vi "2.Réservoir_GJE.vi"() -> ()   [LabVIEW 2018]
panel:
  in  "Consigne":i16(slide) min=0 max=1000 scale=0.0..1000.0
  in  "Débit":i8(slide)=1 min=1 max=10 scale=1.0..10.0
  in  "stop":bool
  out "Tank":i16(slide) scale=0.0..1000.0
  # "1/s"
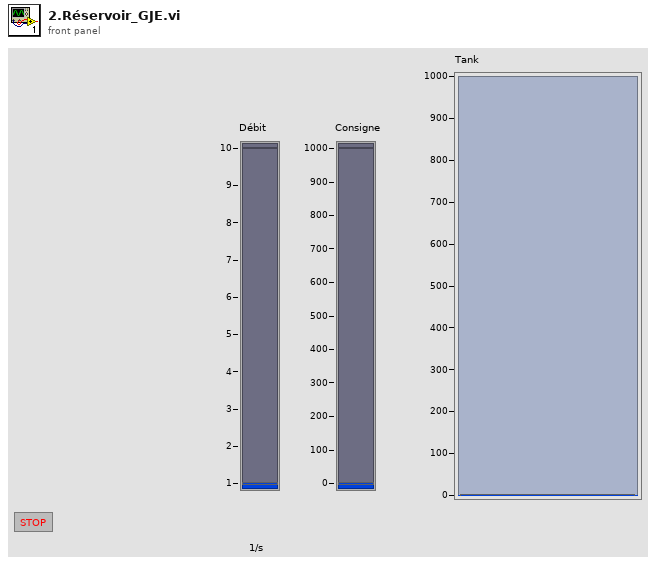
[diagram p1: front panel]
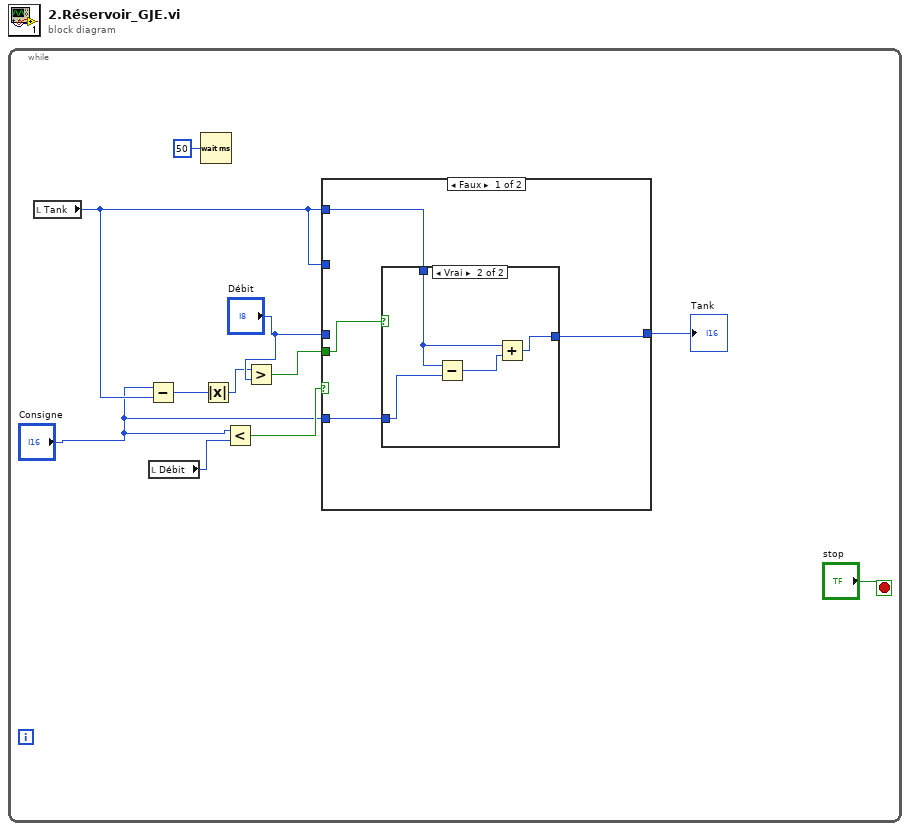
[diagram p0: block diagram]
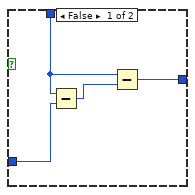
[diagram p2: hidden frame]
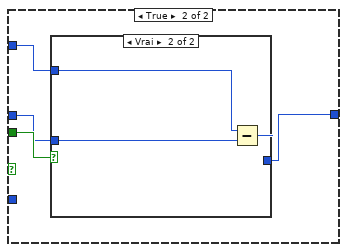
[diagram p3: hidden frame]
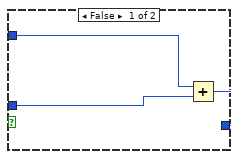
[diagram p4: hidden frame]
diagram:
  n1 = while {
    stop <- "stop" stop-if-true
    n2 = local read "Tank"() -> (w4:i16)
    n3 = Subtract(x="Consigne", y=w4) -> (x-y=w8:i16)
    n4 = local read "Débit"() -> (w1:i8)
    n5 = Wait (ms)(milliseconds to wait=u32 50) -> ()  [unwired: 1 out]
    n6 = Absolute Value(x=w8) -> (abs(x)=w6:i16)
    n7 = Less?(x="Consigne", y=w1) -> (x < y?=w3:bool)
    n8 = Greater?(x=w6, y="Débit") -> (0:w9:bool)
    n9 = case shown="Faux" w3 {
      tunnel: w9 -> [w13 w27]
      tunnel: w4 -> [_ w26]
      tunnel: "Débit" -> [_ w25]
      tunnel: [w12 w24] -> w5
      tunnel: w4 -> [w15 _]
      tunnel: "Consigne" -> [w14 _]
      frame False {
        n10 = case shown="Vrai" w13 {
          tunnel: [w18 w23] -> w12
          tunnel: w15 -> [w16 w21]
          tunnel: w14 -> [w17 w22]
          frame False {
            n11 = Subtract(x=w16, y=w17) -> (x-y=w19:i16)
            n12 = Subtract(x=w16, y=w19) -> (x-y=w18:i16)
          }
          frame True {
            n13 = Subtract(x=w21, y=w22) -> (x-y=w20:i16)
            n14 = Add(x=w21, y=w20) -> (x+y=w23:i16)
          }
        }
      }
      frame True {
        n15 = case shown="Vrai" w27 {
          tunnel: w26 -> [w30 w33]
          tunnel: [w29 w32] -> w24
          tunnel: w25 -> [w28 w31]
          frame False {
            n16 = Add(x=w30, y=w28) -> (x+y=w29:i16)
          }
          frame True {
            n17 = Subtract(x=w33, y=w31) -> (x-y=w32:i16)
          }
        }
      }
    }
    "Tank" <- w5
  }
